vi "TrackTarget.vi"() -> ()   [LabVIEW 2011]
uses:
  Robot Global Data.vi
  <vilib>/addons/control/pid/NI_PID_pid.lvlib
  <vilib>/addons/control/pid/pid.llb/PID (DBL).vi
panel:
  in  "Steer PID gains":T1={"proportional gain (Kc)"=0.05, "integral time (Ti, min)"=0.01, "derivative time (Td, min)"=0.002} {"derivative time (Td, min)" format="%#.7g"; "integral time (Ti, min)" format="%#.6g"; "proportional gain (Kc)" format="%#.6g"}
  in  "saturation":dbl=1.0
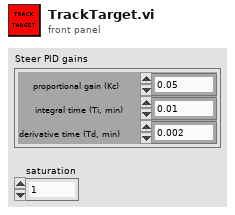
[diagram p1: front panel]
types:
  T1 = cluster{"proportional gain (Kc)":dbl, "integral time (Ti, min)":dbl, "derivative time (Td, min)":dbl}
  T2 = typedef "Position Typedef.ctl" = cluster{"X":dbl, "Y":dbl, "Heading":dbl}
  T3 = typedef "Target Typedef.ctl" = cluster{"X":dbl, "Y":dbl, "Ultrasonic Range (in)":dbl}
  T4 = typedef "WPI_RobotDriveDevRef.ctl" = cluster{"DevStatus":errorcluster, "Motors[]":T5[], "Square Inputs":bool, "Max Output":dbl, "Isochronous":bool}
  T5 = typedef "WPI_MotorControlDeviceRef.ctl" = cluster{"DeviceStatus":errorcluster, "Type":enum16{"PWM", "CAN"}, "PWM":cluster{"Digital Module":T6, "PWM Channel":T7, "DeadBand":T8}, "CAN":cluster{"Device Number":u8, "Control Mode":T9, "Semaphore":T10, "Max Vout":dbl}, "Invert":bool, "TransformRef":T11, "InvTransformRef":T11}
  T6 = typedef "FPGA_TypedefDigitalModule.ctl" = enum16{"Digital Module 1", "Digital Module 2"}
  T7 = typedef "FPGA_DIOPWMChannel.ctl" = enum8{"PWM 1", "PWM 2", "PWM 3", "PWM 4", "PWM 5", "PWM 6", "PWM 7", "PWM 8", "PWM 9", "PWM 10", "Invalid"}
  T8 = typedef "WPI_PWMDeadband.ctl" = cluster{"Name":string, "maxPositivePwm":i32, "minPositivePwm":i32, "centerPwm":i32, "maxNegativePwm":i32, "minNegativePwm":i32, "angularRange":u16}
  T9 = typedef "WPI_CANJaguar_ControlMode.ctl" = enum8{"Percent VBus", "Current", "Speed", "Position", "Voltage"}
  T10 = typedef "Semaphore RefNum" = refnum<k1>
  T11 = typedef "WPI_PWMTransform_ConPane.ctl" = refnum<vi>
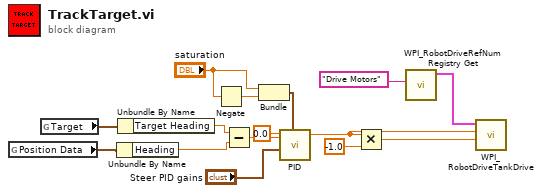
[diagram p0: block diagram]
diagram:
  n1 = global read "Robot Global Data.vi" "Position Data"() -> (w2:T2)
  n2 = global read "Robot Global Data.vi" "Target"() -> (w1:T3)
  n3 = Unbundle By Name(w2) -> ("Heading"=w4:dbl)
  n4 = Unbundle By Name(w1) -> ("Target Heading"=w3:dbl)
  n5 = Negate(x="saturation") -> (-x=w8:dbl)
  n6 = Subtract(x=w3, y=w4) -> (x-y=w5:dbl)
  n7 = Bundle("saturation"="saturation", w8) -> (w9:cluster{"saturation":dbl, dbl})  [unwired: 1 out]
  n8 = call-poly <vilib>:"PID.vi"("output range"=w9, "PID gains"="Steer PID gains", "process variable"=w5, "setpoint"=0.0) -> ("output"=w13:dbl)  [unwired: 6 in, 1 out]
  n9 = Multiply(x=w13, y=-1.0) -> (x*y=w12:dbl)
  n10 = call <vilib>:"WPI_RobotDriveRefNum Registry Get.vi"("refnum name"="Drive Motors") -> ("RobotDriveDevRef"=w15:T4)  [unwired: 1 in, 9 out]
  n11 = call <vilib>:"WPI_RobotDriveTankDrive.vi"("Right axis value"=w12, "Left axis value"=w13, "RobotDriveDevRef"=w15) -> ()  [unwired: 7 in, 2 out]
